vi "AlignStringWithSpaces.vi"(6 "FromBegin":bool, 10 "TargetLength":i32=4, 11 "Input":string) -> (3 "Output":string)   [LabVIEW 2016]
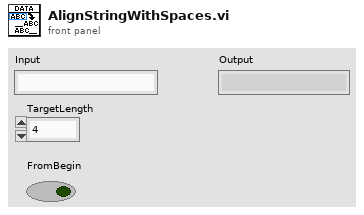
[diagram p1: front panel]
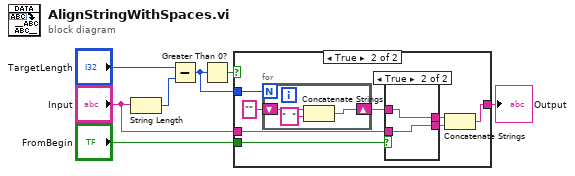
[diagram p0: block diagram]
diagram:
  n1 = String Length(string="Input") -> (length=w7:i32)
  n2 = Subtract(x="TargetLength", y=w7) -> (x-y=w4:i32)
  n3 = Greater Than 0?(x=w4) -> (x > 0?=w5:bool)
  n4 = case shown="True" w5 {
    tunnel: w4 -> [_ w16]
    tunnel: "FromBegin" -> [_ w14]
    tunnel: "Input" -> [w8 w12]
    tunnel: [w8 w9] -> w1
    frame False {
    }
    frame True {
      n5 = for {
        N: w16 -> [_]
        shift-right: [w23] -> w13
        shift-left: "" -> [w22]
        n6 = Concatenate Strings(w22, "  " ("string")) -> (w23:string)
      }
      n7 = case shown="True" w14 {
        tunnel: w13 -> [w17 w20]
        tunnel: w12 -> [w18 w19]
        tunnel: [w18 w20] -> w11
        tunnel: [w17 w19] -> w10
        frame False {
        }
        frame True {
        }
      }
      n8 = Concatenate Strings(w11, w10) -> (w9:string)
    }
  }
  "Output" <- w1
